vi "Gmsg_RR_Sender.vi"() -> ()   [LabVIEW 2013]
uses:
  <vilib>/Math Plots/3D Math Plots/3D Surface/3D Surface XCtrl/3D Surface.xctl
  <vilib>/Analysis/1siggen.llb/Ramp Pattern by Samples.vi
  <vilib>/Math Plots/3D Math Plots/3D Surface/3D Surface Datatype/Public/Plot Helper (Vector).vi
  source/actor/Request/FTW-Request.lvclass
  <vilib>/Analysis/NI_AALBase.lvlib
  <vilib>/Math Plots/3D Math Plots/3D Surface/3D Surface Datatype/3D Surface Datatype.lvclass
panel:
  in  "Response Size":i32=1
  out "Message Roundtrip Times":refnum<class "3D Plot Datatype.lvclass">[](xcontrol)
  in  "Connection":string(combo)="lvq://someLVQconnection"
  out "Histogram Graph":T1(graph)
  out "Shortest Message":dbl format="%#_6p"
  out "Longest Message":dbl format="%#_6p"
  out "Timeout":bool
  in  "Timeout":i32=1000
  out "Timeouts":bool[][](array[boolean])
  in  "Parallel Connections":i32=1
  out "Response Body":string
  in  "Message Size":i32=1
  out "Response Header":string
  out "Avg Msg Roundtrip":dbl format="%#_6p"
  in  "Messages":i32=1
  out "Elapsed":dbl format="%#_6p"
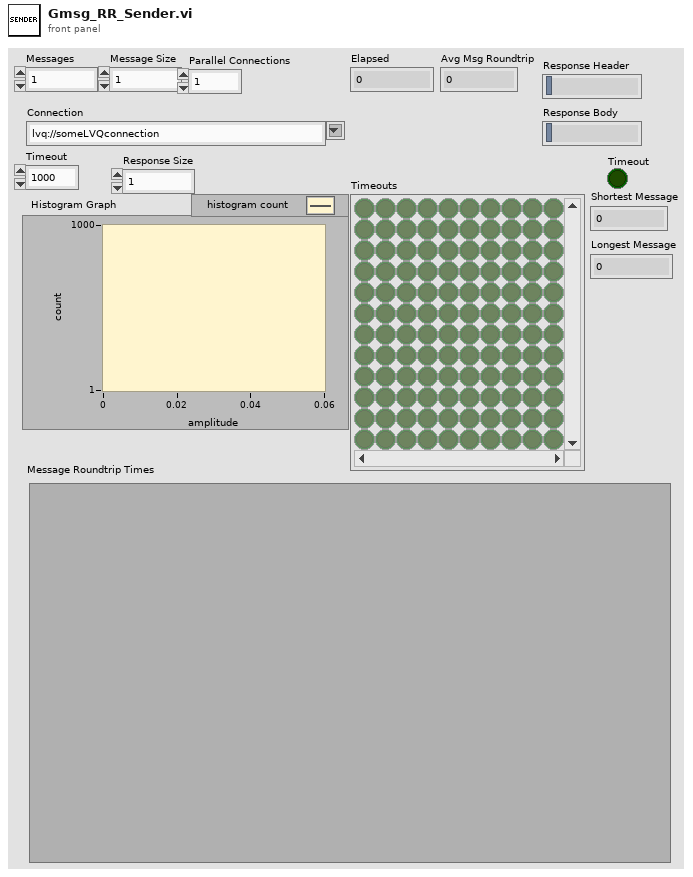
[diagram p1: front panel]
types:
  T1 = cluster{"X Values":dbl[], "Histogram: h(x)":i32[]}
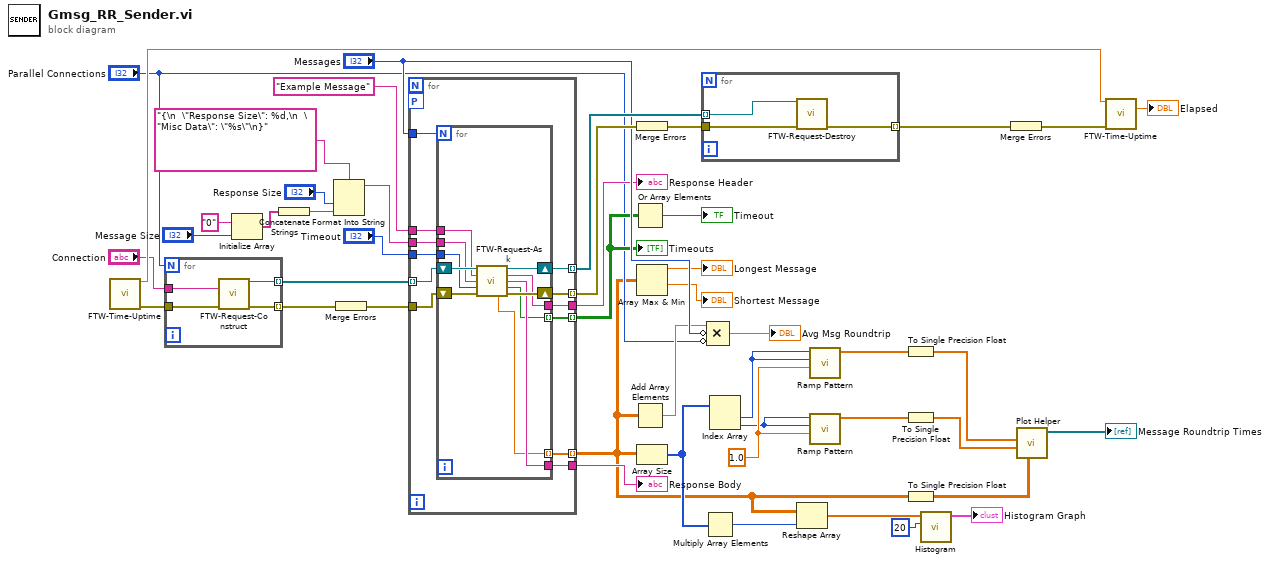
[diagram p0: block diagram]
diagram:
  w14 = 1.0 ("start")
  n1 = call "FTW-Time-Uptime.vi"() -> ("Current Uptime"=w41:dbl, "error out"=w43:errorcluster)  [unwired: 13 in, 1 out]
  n2 = for {
    N: "Parallel Connections" -> [_]
    tunnel: [w50] -> w46 mode=indexing
    tunnel: [w49] -> w45 mode=indexing
    tunnel: w43 -> [w48]
    tunnel: "Connection" -> [w47]
    n3 = call "FTW-Request-Construct.vi"("Server Address"=w47, "error in"=w48) -> ("FTW-Request Out"=w50:refnum<class "FTW-Request.lvclass">, "error out"=w49:errorcluster)  [unwired: 12 in]
  }
  n4 = Initialize Array("0", "Message Size") -> (w32:string[])
  n5 = Concatenate Strings(w32) -> (w3:string)
  n6 = Format Into String(format string="{\n  \"Response Size\": %d,\n  \"Misc Data\": \"%s\"\n}", "Response Size", w3) -> (resulting string=w2:string)  [unwired: 2 in, 1 out]
  n7 = Merge Errors(w45) -> (w21:errorcluster)
  n8 = for {
    tunnel: w46 -> [w62] mode=indexing
    tunnel: [w61] -> w39 mode=indexing
    tunnel: [w60] -> w38 mode=indexing
    tunnel: w21 -> [w59]
    tunnel: "Messages" -> [w58]
    tunnel: "Example Message" ("String") -> [w57]
    tunnel: w2 -> [w56]
    tunnel: [w55] -> w31
    tunnel: [w54] -> w30
    workers-P: _ -> [_]
    tunnel: [w53] -> w26 mode=indexing
    tunnel: "Timeout" -> [w52]
    tunnel: [w51] -> w8 mode=indexing
    n9 = for {
      N: w58 -> [_]
      tunnel: [w67] -> w54
      shift-right: [w70] -> w61
      shift-left: w62 -> [w71]
      shift-right: [w72] -> w60
      shift-left: w59 -> [w73]
      tunnel: w57 -> [w69]
      tunnel: w56 -> [w68]
      tunnel: [w66] -> w55
      tunnel: [w65] -> w53 mode=indexing
      tunnel: w52 -> [w64]
      tunnel: [w63] -> w51 mode=indexing
      n10 = call "FTW-Request-Ask.vi"("FTW-Request In"=w71, "Header"=w69, "Body"=w68, "Timeout"=w64, "error in"=w73) -> ("FTW-Request Out"=w70:refnum<class "FTW-Request.lvclass">, "Response Header"=w66:string, "Response Body"=w67:string, "Timed out?"=w65:bool, "Roundtrip Time"=w63:dbl, "error out"=w72:errorcluster)  [unwired: 5 in]
    }
  }
  "Response Header" <- w31
  "Response Body" <- w30
  "Timeouts" <- w26
  n11 = Or Array Elements(Boolean array=w26) -> (logical OR=→"Timeout":bool)
  n12 = Add Array Elements(numeric array=w8) -> (sum=w22:dbl)
  n13 = Merge Errors(w38) -> (w44:errorcluster)
  n14 = Array Max & Min(array=w8) -> (max value=→"Longest Message":dbl, min value=→"Shortest Message":dbl)  [unwired: 2 out]
  n15 = Array Size(array=w8) -> (size(s)=w15:i32[])
  n16 = for {
    tunnel: w44 -> [w76]
    tunnel: [w75] -> w42 mode=indexing
    tunnel: w39 -> [w74] mode=indexing
    n17 = call "FTW-Request-Destroy.vi"("FTW-Request In"=w74, "error in"=w76) -> ("error out"=w75:errorcluster)  [unwired: 13 in]
  }
  n18 = Multiply Array Elements(1:w15) -> (0:w19:i32)
  n19 = Compound Arithmetic op=MULTIPLY(w22, invert "Messages", invert "Parallel Connections") -> (→"Avg Msg Roundtrip":dbl)
  n20 = Index Array(array=w15) -> (element #1=w12:i32, element #2=w13:i32)  [unwired: 2 in]
  n21 = Reshape Array(w8, w19) -> (w18:dbl[])
  n22 = call-poly <vilib>:"Ramp Pattern.vi"("start"=w14, "end"=w12, "samples"=w12) -> ("Ramp Pattern"=w10:dbl[])  [unwired: 7 in, 1 out]
  n23 = call-poly <vilib>:"Ramp Pattern.vi"("start"=w14, "end"=w13, "samples"=w13) -> ("Ramp Pattern"=w9:dbl[])  [unwired: 7 in, 1 out]
  n24 = To Single Precision Float(number=w10) -> (single precision float=w7:sgl[])
  n25 = To Single Precision Float(number=w9) -> (single precision float=w6:sgl[])
  n26 = To Single Precision Float(number=w8) -> (single precision float=w5:sgl[][])
  n27 = call <vilib>:"Histogram.vi"("intervals"=20, "X"=w18) -> ("Histogram Graph"=→"Histogram Graph":T1)  [unwired: 6 in, 3 out]
  n28 = Merge Errors(w42) -> (w28:errorcluster)
  n29 = call-poly <vilib>:"Plot Helper.vi"("z matrix"=w5, "y vector"=w6, "x vector"=w7) -> ("3D Plot lvclass Array out"=→"Message Roundtrip Times":refnum<class "3D Plot Datatype.lvclass">[])  [unwired: 3 in, 5 out]
  n30 = call "FTW-Time-Uptime.vi"("Previous Uptime"=w41, "error in"=w28) -> ("Elapsed Time"=→"Elapsed":dbl)  [unwired: 11 in, 2 out]
